vi "ABR-Filter.vi"(0 "ABR raw":dbl[](array[numeric]), 7 "sampling freq: fs":dbl=25000.0 format="%0.2f", 11 "error in (no error)":errorcluster) -> (4 "ABR filtered":dbl[](array[numeric]), 15 "error out":errorcluster)   [LabVIEW 2020]
uses:
  <vilib>/Analysis/3filter.llb/Filter Passband Type.ctl
  <vilib>/Analysis/3filter.llb/Filter Structure Type.ctl
  <vilib>/Analysis/3filter.llb/Zero Phase Filter (Cascade, DBL).vi
  <vilib>/Analysis/NI_AALBase.lvlib
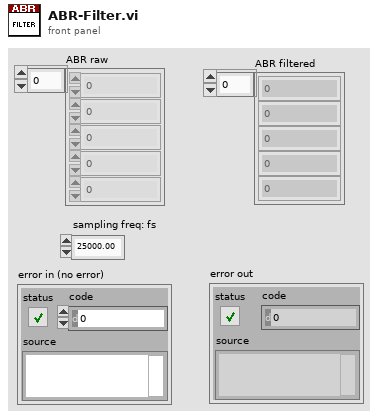
[diagram p1: front panel]
types:
  T1 = typedef "NI_AALBase.lvlib/Filter Structure Type.ctl" = u16
  T2 = typedef "NI_AALBase.lvlib/Filter Passband Type.ctl" = enum32{"Lowpass", "Highpass", "Bandpass", "Bandstop"}
  T3 = cluster{"filter structure":enum32{"IIR 2nd Order", "IIR 4th Order"}, "Reverse Coefficients":dbl[], "Forward Coefficients":dbl[]}
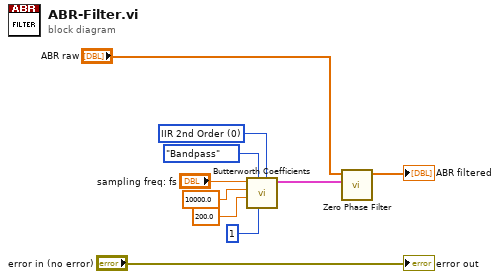
[diagram p0: block diagram]
diagram:
  w8 = T1 0 items=["IIR 2nd Order"=0, "IIR 4th Order"=1, "Auto Select"=10] ("filter structure option")
  n1 = call <vilib>:"Butterworth Coefficients.vi"("filter structure option"=w8, "order"=1, "filter type"=Filter_Passband_Type."Bandpass", "low cutoff freq: fl"=200.0, "high cutoff freq: fh"=10000.0, "sampling freq: fs"="sampling freq: fs") -> ("IIR Filter Cluster"=w3:T3)  [unwired: 4 in, 1 out]
  n2 = call-poly <vilib>:"Zero Phase Filter.vi"("IIR Filter Cluster"=w3, "X"="ABR raw") -> ("Filtered X"=→"ABR filtered":dbl[])  [unwired: 8 in, 1 out]
  "error out" <- "error in (no error)"
